vi "Write State.vi"(8 "error in (no error)":errorcluster, 10 "State":refnum<class "State Pattern.lvclass">, 11 "A Context State in":refnum<class "A Context State.lvclass">) -> (0 "error out":errorcluster, 3 "A Context State out":refnum<class "A Context State.lvclass">)   [LabVIEW 2021, in "Context Actor.lvlib" / "A Context State.lvclass"]
uses:
  A Context State.lvclass
  State Pattern/State Pattern.lvclass
  A Context State.lvclass/A Context State.ctl
  Context Actor.lvclass
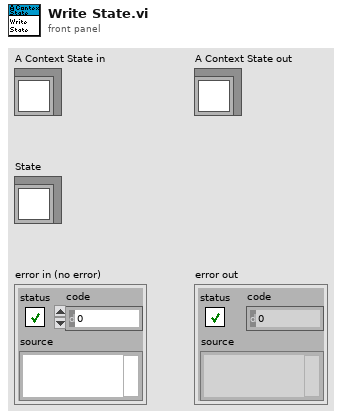
[diagram p1: front panel]
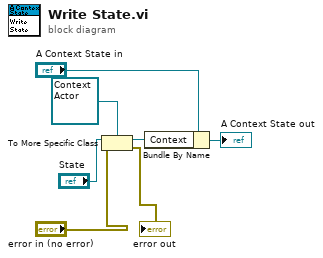
[diagram p0: block diagram]
diagram:
  n1 = To More Specific Class(target class=refnum<class "Context Actor.lvclass"> refnum ("Context Actor.lvlib:Context Actor.lvclass"), reference="State", error in="error in (no error)") -> (specific class reference=w2:refnum<class "Context Actor.lvclass">, error out=→"error out":errorcluster)
  n2 = Bundle By Name(cluster="A Context State in", "Context"=w2) -> (→"A Context State out":refnum<class "A Context State.lvclass">)
